vi "GLIMPSE Get N and Y.vi"(4 "Y In (Phys)":u32, 5 "# of Frames In (Phys)":u32, 7 "Frame # In (Log)":u32) -> (0 "Y Out (Log)":u32, 1 "# of Frames Out (Log)":u32, 3 "Frame # Out (Phys)":u32)   [LabVIEW 2011]
uses:
  GLIMPSE Globals.vi
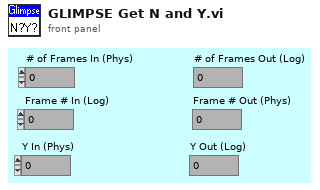
[diagram p1: front panel]
types:
  T1 = enum16{"Frames", "Fields, Odd 1st", "Fields, Even 1st", "Fields, Averaged"}
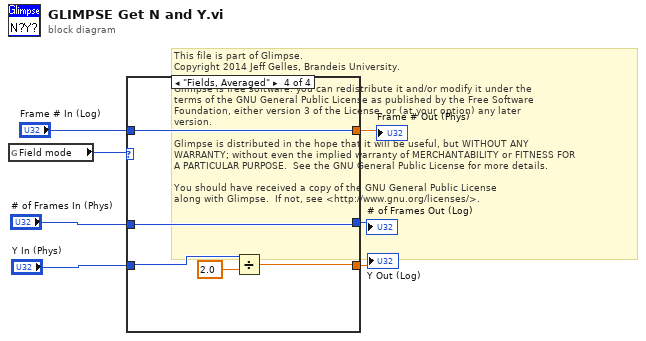
[diagram p0: block diagram]
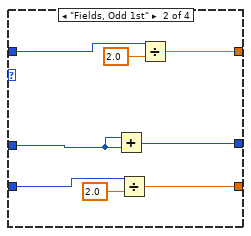
[diagram p3: hidden frame]
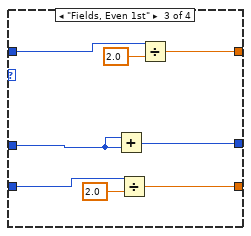
[diagram p4: hidden frame]
diagram:
  # "This file is part of Glimpse. \nCopyright 2014 Jeff Gelles, Brandeis University.    \n\nGlimpse is free software: you can redistribute it and/or modify it under the \nterms of the GNU General Public License as published by the Free Software \nFoundation, either version 3 of the License, or (at your option) any later \nversion.\n\nGlimpse is distributed in the hope that it will be useful, but WITHOUT ANY \nWARRANTY; without even the implied warranty of MERCHANTABILITY or FITNESS FOR \nA PARTICULAR PURPOSE.  See the GNU General Public License for more details.\n\nYou should have received a copy of the GNU General Public License\nalong with Glimpse.  If not, see <http://www.gnu.org/licenses/>."
  n1 = global read "GLIMPSE Globals.vi" "Field mode"() -> (w1:T1)
  n2 = case shown="\"Fields, Averaged\"" w1 {
    tunnel: "# of Frames In (Phys)" -> [w10 w18 w26 w30]
    tunnel: [w10 w17 w25 w30] -> w6
    tunnel: "Y In (Phys)" -> [w9 w15 w23 w28]
    tunnel: [w9 w14 w22 w27] -> w4
    tunnel: "Frame # In (Log)" -> [w8 w12 w20 w31]
    tunnel: [w8 w11 w19 w31] -> w2
    frame "Frames" {
    }
    frame "Fields, Odd 1st" {
      n3 = Add(x=w18, y=w18) -> (x+y=w17:u32)
      n4 = Divide(x=w15, y=2.0) -> (x/y=w14:dbl)
      n5 = Divide(x=w12, y=2.0) -> (x/y=w11:dbl)
    }
    frame "Fields, Even 1st" {
      n6 = Add(x=w26, y=w26) -> (x+y=w25:u32)
      n7 = Divide(x=w23, y=2.0) -> (x/y=w22:dbl)
      n8 = Divide(x=w20, y=2.0) -> (x/y=w19:dbl)
    }
    frame "Fields, Averaged" {
      n9 = Divide(x=w28, y=2.0) -> (x/y=w27:dbl)
    }
  }
  "# of Frames Out (Log)" <- w6
  "Y Out (Log)" <- w4
  "Frame # Out (Phys)" <- w2
